vi "Copy files.vi"() -> ()   [LabVIEW 2016]
uses:
  <vilib>/Utility/sysdir.llb/System Directory Type.ctl
panel:
  out "error out":errorcluster
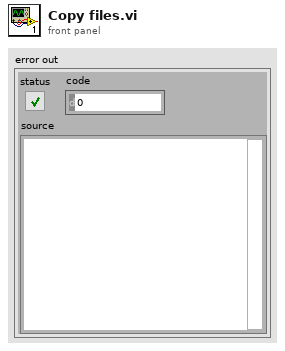
[diagram p1: front panel]
types:
  T1 = typedef "System Directory Type.ctl" = i32
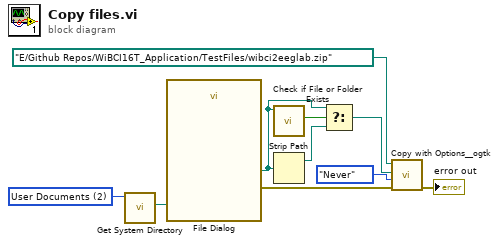
[diagram p0: block diagram]
diagram:
  w7 = T1 2 items=["User Home"=0, "User Desktop"=1, "User Documents"=2, "User Application Data"=3, "User Preferences"=4, "User Temporary"=5, "Public Documents"=6, "Public Application Data"=7, "Public Preferences"=8, "Public Cache"=13, "System Core Libraries"=9, "System Installed Libraries"=10, "Application Files"=11, "Boot Volume Root"=12] ("system directory type")
  n1 = call <vilib>:"Get System Directory.vi"("system directory type"=w7) -> ("system directory"=w6:path)  [unwired: 10 in]
  n2 = call "File Dialog"("start path"=w6) -> ("selected path"=w4:path, "error out"=w1:errorcluster)  [unwired: 11 in, 2 out]
  n3 = call <vilib>:"Check if File or Folder Exists.vi"("path"=w4) -> ("file or folder exists?"=w5:bool)  [unwired: 8 in, 2 out]
  n4 = Strip Path(path=w4) -> (stripped path=w3:path)  [unwired: 1 out]
  n5 = Select(t=w4, s=w5, f=w3) -> (s? t:f=w2:path)
  n6 = call <userlib>:"Copy with Options__ogtk.vi"("error in (no error)"=w1, "Replace Mode (Never)"=enum16{"Never", "Always", "If Newer"}."Never", "target path"=w2, "source path"=path "E:/Github Repos/WiBCI16T_Application/TestFiles/wibci2eeglab.zip" ("selected path")) -> ("error out"=→"error out":errorcluster)  [unwired: 6 in, 1 out]
